vi "Calc Eval.vi"(8 "error in (no error)":errorcluster, 10 "Inputs":dbl[](array[numeric]), 11 "Div Calc in":refnum<class "Div Calc.lvclass">) -> (0 "error out":errorcluster, 1 "Additional Updates":T1[](array[typedef]), 2 "Result":dbl, 3 "Div Calc out":refnum<class "Div Calc.lvclass">)   [LabVIEW 2020, in "VolatusCalcs.lvlib" / "Div Calc.lvclass"]
uses:
  Div Calc.lvclass
  Div Calc.lvclass/Div Calc.ctl
  Calculation/Additional Update.ctl
  Calculation/Calculation.lvclass
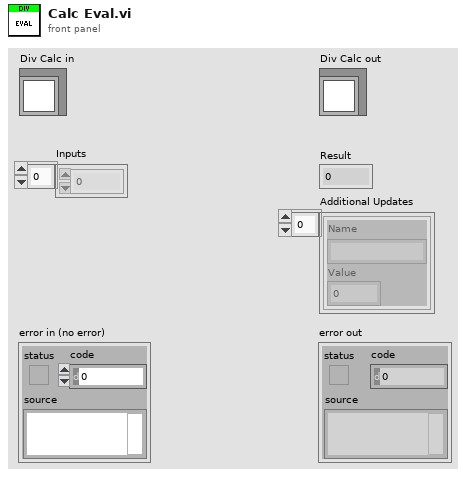
[diagram p1: front panel]
types:
  T1 = typedef "VolatusCalcs.lvlib/Calculation.lvclass/Additional Update.ctl" = cluster{"Name":string, "Value":dbl}
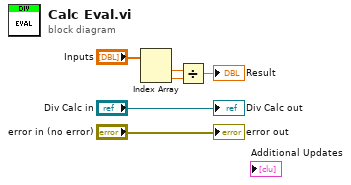
[diagram p0: block diagram]
diagram:
  n1 = Index Array(array="Inputs") -> (element #1=w3:dbl, element #2=w2:dbl)  [unwired: 2 in]
  n2 = Divide(x=w3, y=w2) -> (x/y=→"Result":dbl)
  "error out" <- "error in (no error)"
  "Div Calc out" <- "Div Calc in"
